vi "Error Handler - Message Handling Loop.vi"(8 "error in (no error)":errorcluster caption="错误输入（无错误）", 10 "Ignore Errors (Runtime)":i32[](array[numeric]) caption="忽略错误（运行时）", 11 "Message Queue":refnum<queue> caption="消息队列") -> (0 "dup error in":errorcluster caption="错误输入副本", 3 "dup Message Queue":refnum<queue> caption="消息队列副本")   [LabVIEW 2014]
doc: "对“消息处理循环”中出现的错误进行处理：忽略该错误，或者为该错误生成一个Error消息。"
uses:
  Message Queue/Message Cluster.ctl
  Message Queue/Message Queue.lvlib
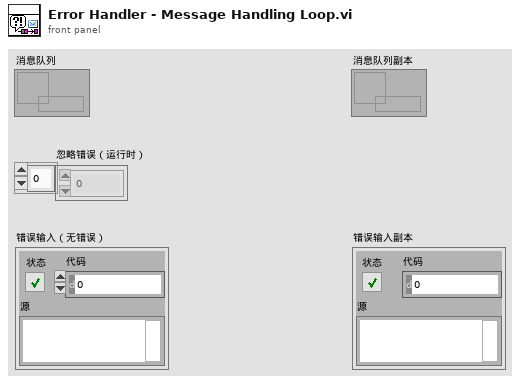
[diagram p1: front panel]
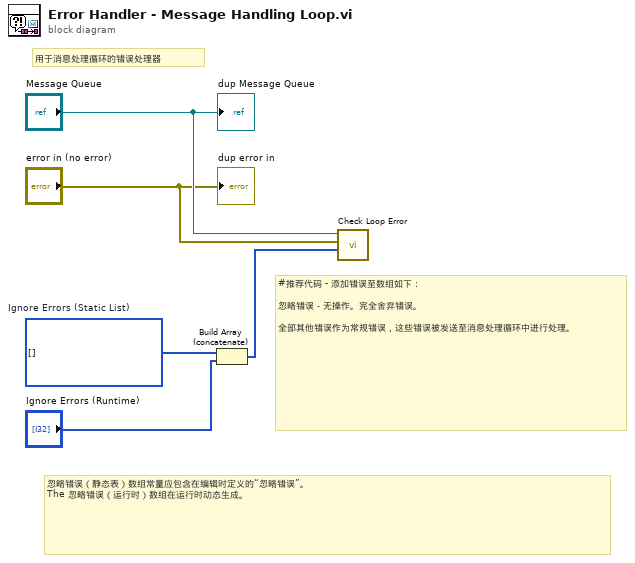
[diagram p0: block diagram]
diagram:
  w3 = i32[] []  # Ignore Errors (Static List)
  # "忽略错误（静态表）数组常量应包含在编辑时定义的“忽略错误”。\nThe 忽略错误（运行时）数组在运行时动态生成。"
  # "#推荐代码 - 添加错误至数组如下：\n\n忽略错误－无操作。完全舍弃错误。\n\n全部其他错误作为常规错误，这些错误被发送至消息处理循环中进行处理。"
  # "用于消息处理循环的错误处理器"
  n1 = Build Array (concatenate)(w3, "Ignore Errors (Runtime)") -> (w1:i32[])
  n2 = call "Check Loop Error.vi"("Ignore Errors"=w1, "error to process"="error in (no error)", "Message Queue"="Message Queue") -> ()  [unwired: 7 in, 2 out]
  "dup Message Queue" <- "Message Queue"
  "dup error in" <- "error in (no error)"
